vi "GetErrorMessageBoxFromDLL.vi"(8 "error IN":errorcluster) -> (0 "error OUT":errorcluster)   [LabVIEW 2020]
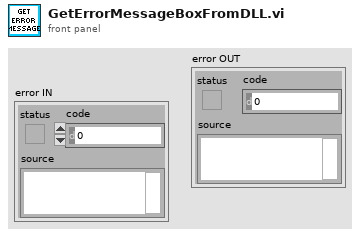
[diagram p1: front panel]
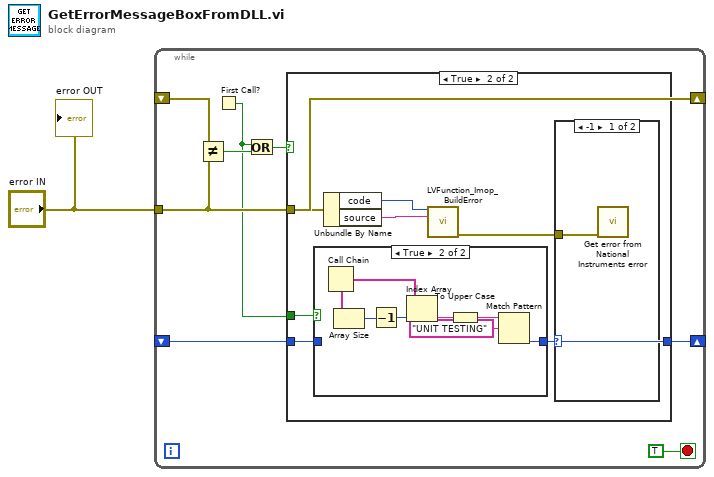
[diagram p0: block diagram]
diagram:
  n1 = while {
    tunnel: "error IN" -> [w8]
    shift-right: [w8] -> _
    shift-left: _ -> [w9]
    shift-right: [w3] -> _
    shift-left: _ -> [w2]
    stop <- TRUE stop-if-true
    n2 = Not Equal?(x=w9, y=w8) -> (x != y?=w6:bool)
    n3 = First Call?() -> (First Call?: T/F=w4:bool)
    n4 = Or(x=w4, y=w6) -> (x .or. y?=w5:bool)
    n5 = case shown="True" w5 {
      tunnel: w8 -> [_ w15]
      tunnel: w4 -> [_ w13]
      tunnel: [w10 w12] -> w3
      tunnel: w2 -> [w10 w11]
      frame False {
      }
      frame True {
        n6 = case shown="True" w13 {
          tunnel: [w18 w19] -> w12
          tunnel: w11 -> [w18 _]
          frame False {
          }
          frame True {
            n7 = Call Chain() -> (call chain=w25:string[])
            n8 = Array Size(array=w25) -> (size(s)=w24:i32)
            n9 = Decrement(x=w24) -> (x-1=w23:i32)
            n10 = Index Array(array=w25, index=w23) -> (element=w22:string)
            n11 = To Upper Case(1:w22) -> (0:w21:string)
            n12 = Match Pattern(string=w21, regular expression="UNIT TESTING") -> (offset past match=w19:i32)  [unwired: 1 in, 3 out]
          }
        }
        n13 = Unbundle By Name(w15) -> ("code"=w17:i32, "source"=w16:string)
        n14 = call "LVFunction_Imop_BuildError.vi"("code"=w17, "String to Prepend to source (\"\")"=w16) -> ("error out"=w14:errorcluster)  [unwired: 13 in]
        n15 = case shown="-1" w12 {
          tunnel: w14 -> [w26 _]
          frame -1 {
            n16 = call "Get error from National Instruments error.vi"("error out"=w26) -> ()  [unwired: 15 in]
          }
          frame 0, Default {
          }
        }
      }
    }
  }
  "error OUT" <- "error IN"
